vi "Get_Active User Layer.vi"(8 "error in (no error)":errorcluster, 11 "Icon in":refnum<class "Icon.lvclass">) -> (0 "error out":errorcluster, 2 "Layer.lvclass":refnum<class "Layer.lvclass">, 3 "Icon out":refnum<class "Icon.lvclass">)   [LabVIEW 2020, in "Icon.lvclass"]
doc: "Return the active User Layer"
uses:
  Icon.lvclass
  Layer/Layer.lvclass
  Icon.lvclass/Icon.ctl
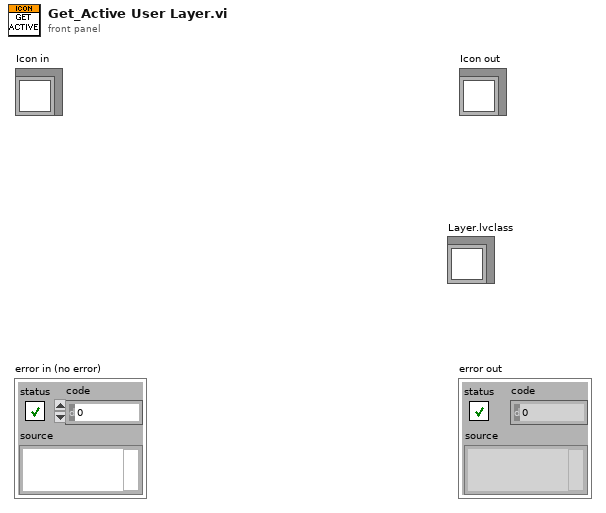
[diagram p1: front panel]
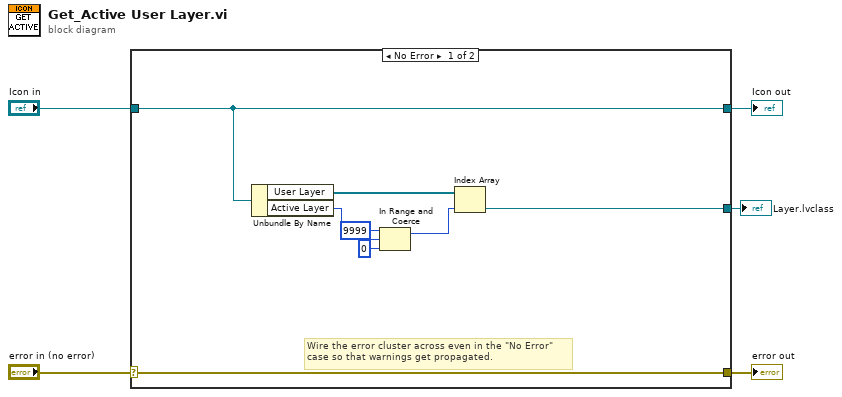
[diagram p0: block diagram]
diagram:
  n1 = case shown="No Error" "error in (no error)" {
    selector: "error in (no error)" -> [w13 w15]
    tunnel: [w13 w15] -> w4
    tunnel: [w12 w14] -> w2
    tunnel: "Icon in" -> [w12 w14]
    tunnel: [w6 _] -> w1
    frame No Error {
      # "Wire the error cluster across even in the \"No Error\"\ncase so that warnings get propagated."
      n2 = Unbundle By Name(w12) -> ("User Layer"=w8:refnum<class "Layer.lvclass">[], "Active Layer"=w11:i32)
      n3 = In Range and Coerce(upper limit=9999, x=w11, lower limit=0) -> (coerced(x)=w7:i32)  [unwired: 1 out]
      n4 = Index Array(array=w8, index=w7) -> (element=w6:refnum<class "Layer.lvclass">)
    }
    frame Error {
    }
  }
  "error out" <- w4
  "Icon out" <- w2
  "Layer.lvclass" <- w1
